vi "Config Timer App.vi"() -> ()   [LabVIEW 2017]
uses:
  subVIs/ModeEnumControl.ctl
  subVIs/AlarmElementControl.ctl
  subVIs/StateEnum.ctl
  subVIs/ModeEnum.ctl
  subVIs/AvailableEnum.ctl
  subVIs/StopWatchTimerStateEnum.ctl
  subVIs/AlarmConvertDirectionEnumControl.ctl
  subVIs/TimerActionEnumControlFGV.ctl
  <vilib>/Utility/file.llb/Write Delimited Spreadsheet (string).vi
  <vilib>/Utility/file.llb/Read Delimited Spreadsheet (string).vi
panel:
  out "Alarm Name":string
  out "Alarm":bool
  out "Path":path
  in  "stop":bool
  out "error out":errorcluster
  out "Clock":string
  in  "Mode Tabs":T1
  in  "Alarm Edit":bool
  in  "Alarm Save":bool
  in  "Alarm List":T2[](array[typedef])
  out "Timer Error":errorcluster
  out "Expired":bool
  out "Elasped Time":i32
  in  "Timer Start/Stop":bool
  in  "Duration (s)":i32
  in  "Lap":bool
  in  "Pause":bool
  out "SW Elapsed Time (s)":dbl format="%.1g"
  in  "SW Timer Start/Stop":bool
  out "SW Error":errorcluster
  # "(one at a time)"
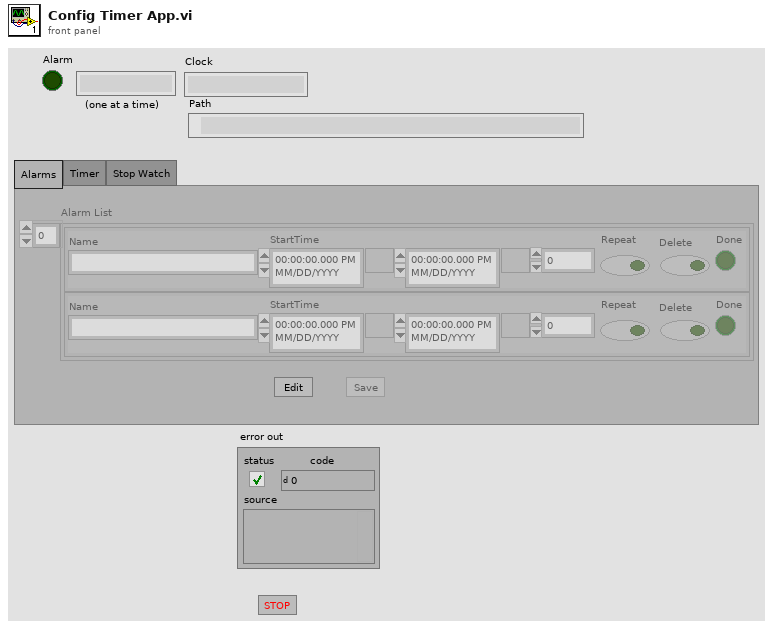
[diagram p1: front panel]
types:
  T1 = typedef "ModeEnumControl.ctl" = enum32{"Alarms", "Timer", "Stop Watch"}
  T2 = typedef "AlarmElementControl.ctl" = cluster{"Name":string, "StartTime ":timestamp, "End Time":timestamp, "Duration":i32, "Repeat":bool, "Delete":bool, "Done":bool}
  T3 = typedef "StopWatchTimerStateEnum.ctl" = enum16{"Start", "Idle", "Timing", "Lap", "Pause", "Stop"}
  T4 = cluster{"State":T3, "Duration":i32, "Start/Stop":bool, "Elapsed Time":dbl, "Expired":bool, "Pause":bool, "Lap":bool}
  T5 = cluster{"State":T3, "Duration":i32, "Start/Stop":bool, "Elapsed Time":i32, "Expired":bool}
  T6 = typedef "StateEnum.ctl" = enum16{"Startup", "Read Config", "Idle", "Timer"}
  T7 = typedef "ModeEnum.ctl" = enum16{"Alarms", "Timer"}
  T8 = typedef "AvailableEnum.ctl" = enum8{"Enabled", "Disabled", "Disabled and Grayed Out"}
  T9 = cluster{"State":T6, "Mode":T7, "Alarms":T2[], "Time":timestamp, "Alarm Edit Flag":bool, "Alarm List and Save Status":T8, "Alarm Edit Status":T8, "Path":path, "File":string, "Alarm Flag":bool, "Alarm Index":i32, "Alarmed Already":bool}
  T10 = typedef "TimerActionEnumControlFGV.ctl" = enum16{"Reset", "TimeQuery", "Pause", "Unpause"}
  T11 = typedef "AlarmConvertDirectionEnumControl.ctl" = enum16{"ToString", "ToCluster"}
  T12 = typedef "LVDateTimeRec.ctl" = cluster{"fractional second":dbl, "second":i32, "minute":i32, "hour":i32, "day of month":i32, "month":i32, "year":i32, "day of week":i32, "day of year":i32, "DST":i32}
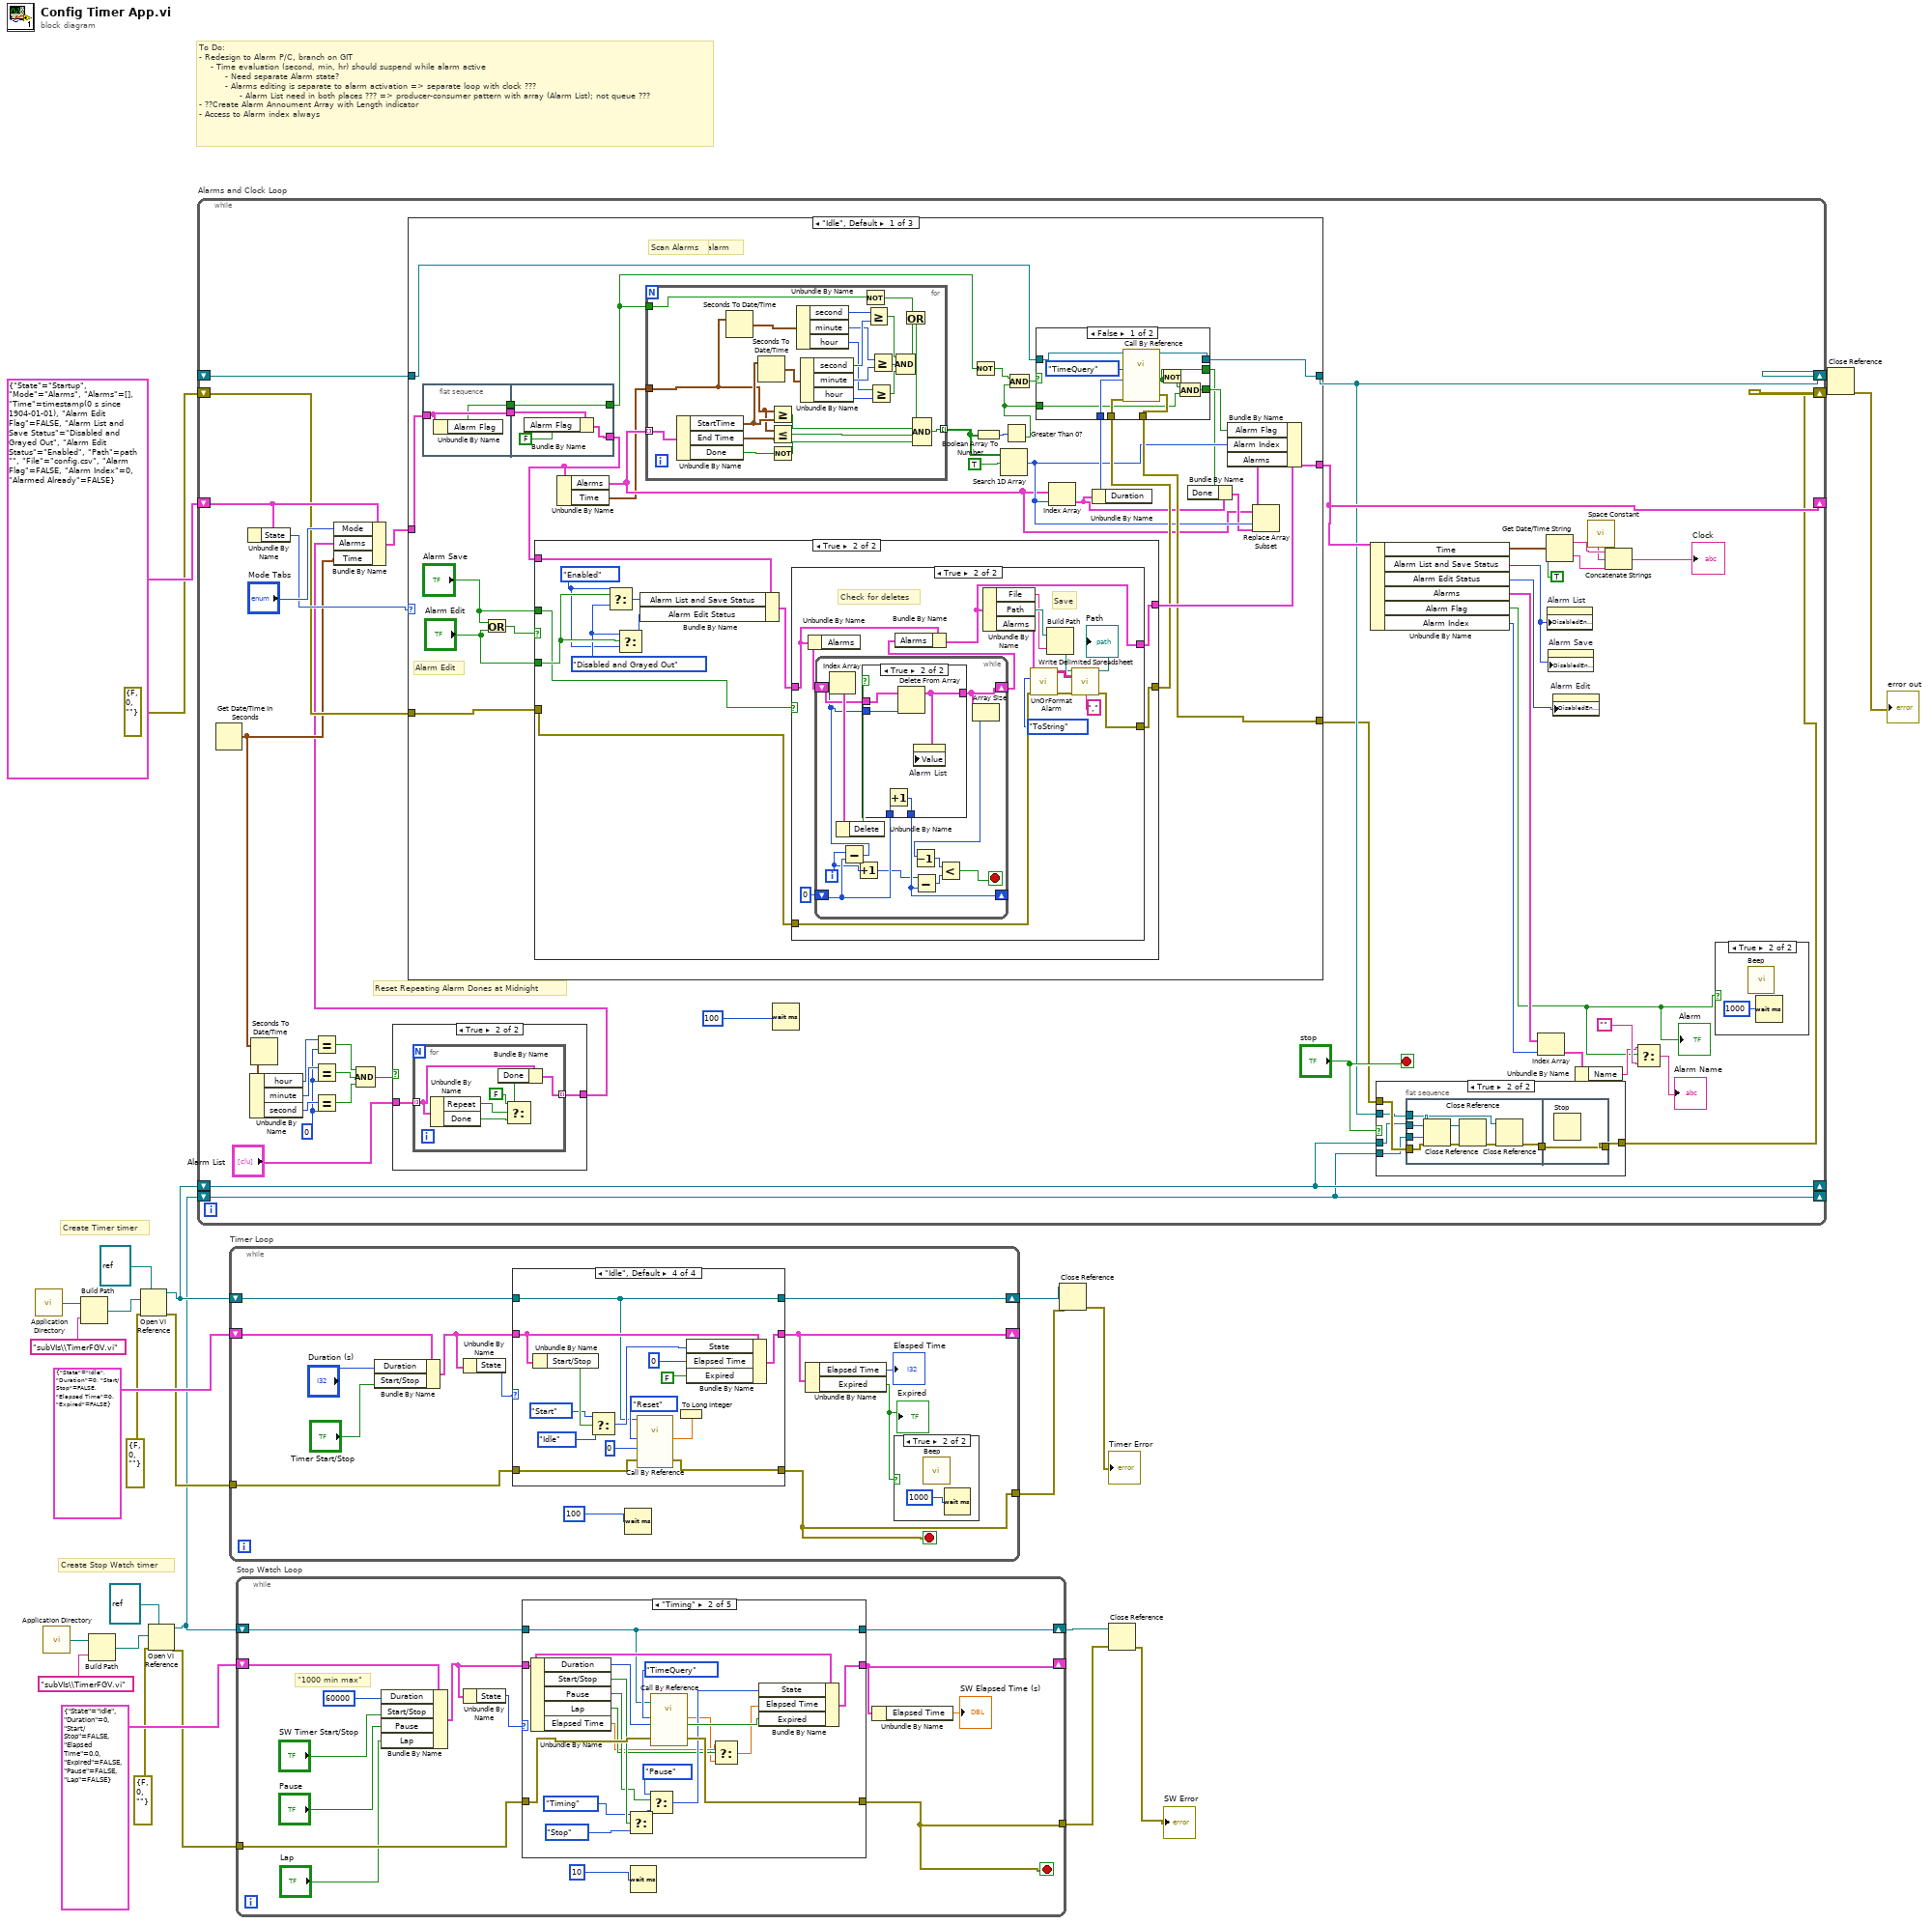
[diagram p0: block diagram]
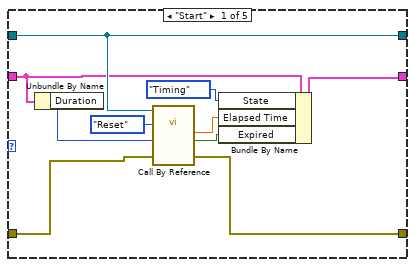
[diagram p2: hidden frame]
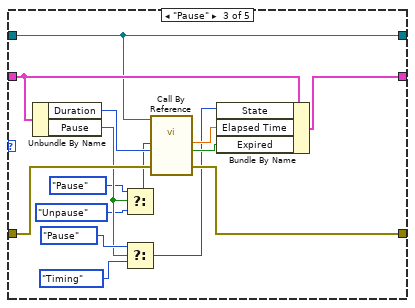
[diagram p3: hidden frame]
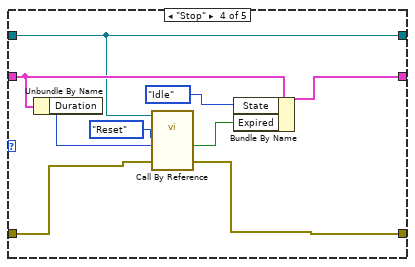
[diagram p4: hidden frame]
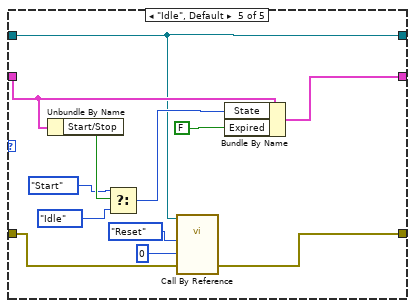
[diagram p5: hidden frame]
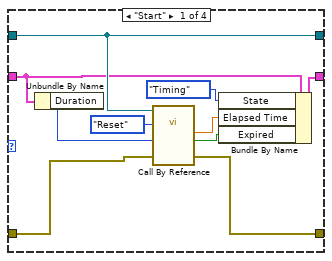
[diagram p7: hidden frame]
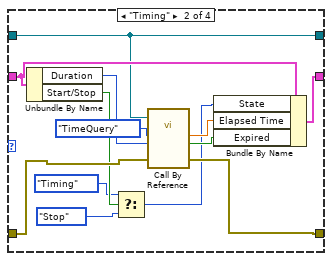
[diagram p8: hidden frame]
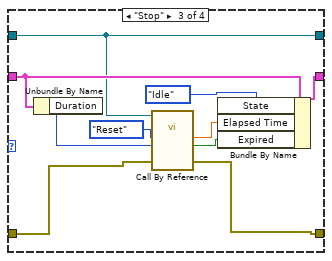
[diagram p9: hidden frame]
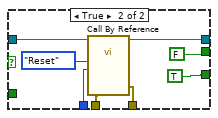
[diagram p13: hidden frame]
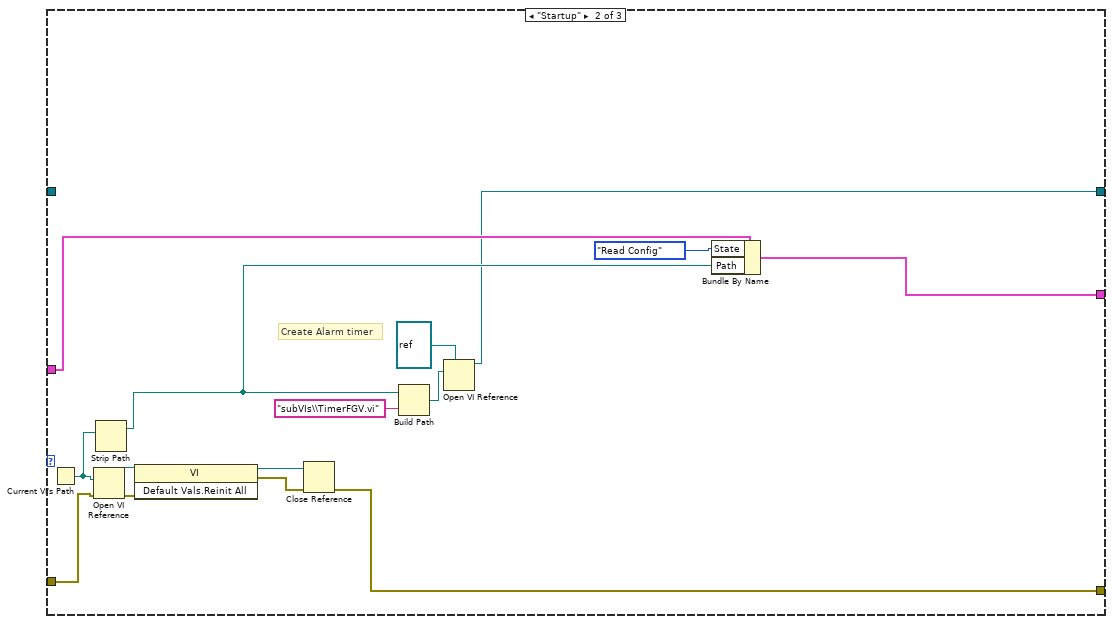
[diagram p17: hidden frame]
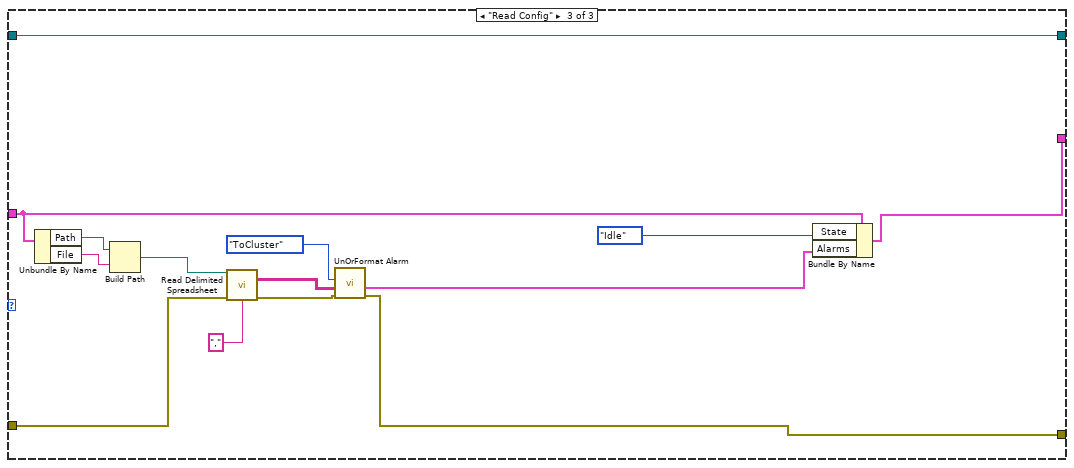
[diagram p18: hidden frame]
diagram:
  # "Create Stop Watch timer"
  # "Create Timer timer"
  # "To Do:\n- Redesign to Alarm P/C, branch on GIT\n    - Time evaluation (second, min, hr) should suspend while alarm active\n         - Need separate Alarm state?\n         - Alarms editing is separate to alarm activation => separate loop with clock ??? \n              - Alarm List need in both places ??? => producer-consumer pattern with array (Alarm List); not queue ???\n- ??Create Alarm Annoument Array with Length indicator\n- Access to Alarm index always"
  n1 = call <vilib>:"Application Directory.vi"() -> ("Application Directory"=w24:path)
  n2 = call <vilib>:"Application Directory.vi"() -> ("Application Directory"=w21:path)
  n3 = Build Path(base path=w24, name or relative path="subVIs\\TimerFGV.vi") -> (appended path=w18:path)
  n4 = Build Path(base path=w21, name or relative path="subVIs\\TimerFGV.vi") -> (appended path=w14:path)
  n5 = Open VI Reference(type specifier VI Refnum (for type only)=refnum<vi> refnum, vi path=w18, error in (no error)=errorcluster {"status"=FALSE, "code"=0, "source"=""} ("error constant")) -> (vi reference=w11:refnum<vi>, error out=w16:errorcluster)  [unwired: 3 in]
  n6 = Open VI Reference(type specifier VI Refnum (for type only)=refnum<vi> refnum, vi path=w14, error in (no error)=errorcluster {"status"=FALSE, "code"=0, "source"=""} ("error constant")) -> (vi reference=w10:refnum<vi>, error out=w12:errorcluster)  [unwired: 3 in]
  n7 = while "Alarms and Clock Loop" {
    shift-right: [w62] -> _
    shift-left: T9 {"State"=enum."Startup", "Mode"=enum."Alarms", "Alarms"=[], "Time"=timestamp(0 s since 1904-01-01), "Alarm Edit Flag"=FALSE, "Alarm List and Save Status"=enum."Disabled and Grayed Out", "Alarm Edit Status"=enum."Enabled", "Path"=path "", "File"="config.csv", "Alarm Flag"=FALSE, "Alarm Index"=0, "Alarmed Already"=FALSE} -> [w67]
    shift-right: [w29] -> w2
    shift-left: errorcluster {"status"=FALSE, "code"=0, "source"=""} ("error constant") -> [w64]
    shift-right: [w31] -> w4
    shift-left: _ -> [w51]
    shift-right: [w33] -> _
    shift-left: w11 -> [w33]
    shift-right: [w32] -> _
    shift-left: w10 -> [w32]
    stop <- "stop" stop-if-true
    w35 = 0
    # "Reset Repeating Alarm Dones at Midnight"
    n8 = Get Date/Time In Seconds() -> (seconds since 1Jan1904=w46:timestamp)
    n9 = Unbundle By Name(w67) -> ("State"=w65:T6)
    n10 = Seconds To Date/Time(time stamp (now)=w46) -> (date time rec=w45:T12)  [unwired: 1 in]
    n11 = Unbundle By Name(w45) -> ("hour"=w36:i32, "minute"=w44:i32, "second"=w43:i32)
    n12 = Equal?(x=w36, y=w35) -> (x = y?=w40:bool)
    n13 = Equal?(x=w44, y=w35) -> (x = y?=w41:bool)
    n14 = Equal?(x=w43, y=w35) -> (x = y?=w42:bool)
    n15 = Compound Arithmetic op=AND(w40, w41, w42) -> (w39:bool)
    n16 = case shown="True" w39 {
      tunnel: "Alarm List" -> [w85 w87]
      tunnel: [w85 w86] -> w37
      frame False {
      }
      frame True {
        n17 = for {
          tunnel: w87 -> [w92] mode=indexing
          tunnel: [w93] -> w86 mode=indexing
          n18 = Unbundle By Name(w92) -> ("Repeat"=w91:bool, "Done"=w89:bool)
          n19 = Select(t=FALSE, s=w91, f=w89) -> (s? t:f=w88:bool)
          n20 = Bundle By Name(cluster=w92, "Done"=w88) -> (w93:T2)
        }
      }
    }
    n21 = Bundle By Name(cluster=w67, "Mode"="Mode Tabs", "Alarms"=w37, "Time"=w46) -> (w63:T9)
    n22 = case shown="\"Idle\", Default" w65 {
      tunnel: w64 -> [w120 w235 w240]
      tunnel: [w110 w232 w239] -> w30
      tunnel: w63 -> [w109 w226 w249]
      tunnel: [w118 w230 w250] -> w62
      tunnel: [w113 w223 w238] -> w31
      tunnel: w51 -> [w114 _ w238]
      frame "Idle", Default {
        # "Find only first alarm"
        # "Alarm Edit"
        # "Scan Alarms"
        n23 = flat-sequence {
          tunnel: w109 -> [w143]
          tunnel: [w143] -> w107
          tunnel: [w142] -> w105
          tunnel: [w146] -> w108
          tunnel: w107 -> [w145]
          tunnel: [w144] -> w94
          tunnel: w105 -> [w144]
          frame #0 {
            n24 = Unbundle By Name(w143) -> ("Alarm Flag"=w142:bool)
          }
          frame #1 {
            n25 = Bundle By Name(cluster=w145, "Alarm Flag"=FALSE) -> (w146:T9)
          }
        }
        n26 = Or(x="Alarm Save", y="Alarm Edit") -> (x .or. y?=w123:bool)
        n27 = case shown="True" w123 {
          tunnel: w108 -> [w173 w184]
          tunnel: [w173 w174] -> w119
          tunnel: "Alarm Edit" -> [_ w183]
          tunnel: "Alarm Save" -> [_ w178]
          tunnel: w120 -> [w172 w176]
          tunnel: [w172 w175] -> w111
          frame False {
          }
          frame True {
            w181 = AvailableEnum."Disabled and Grayed Out" ("Enum")
            w180 = AvailableEnum."Enabled" ("Enum")
            n28 = Select(t=w180, s=w183, f=w181) -> (s? t:f=w182:T8)
            n29 = Select(t=w181, s=w183, f=w180) -> (s? t:f=w179:T8)
            n30 = Bundle By Name(cluster=w184, "Alarm List and Save Status"=w182, "Alarm Edit Status"=w179) -> (w177:T9)
            n31 = case shown="True" w178 {
              tunnel: w177 -> [w185 w191]
              tunnel: w176 -> [w186 w201]
              tunnel: [w186 w195] -> w175
              tunnel: [w185 w189] -> w174
              frame False {
              }
              frame True {
                # "Check for deletes"
                # "Save"
                n32 = Unbundle By Name(w191) -> ("Alarms"=w190:T2[])
                n33 = while {
                  shift-right: [w208] -> _
                  shift-left: 0 -> [w206]
                  shift-right: [w203] -> w187
                  shift-left: w190 -> [w213]
                  i -> [w205]
                  stop <- w210 stop-if-true
                  n34 = Subtract(x=w205, y=w206) -> (x-y=w209:i32)
                  n35 = Index Array(array=w213, index=w209) -> (element=w215:T2)
                  n36 = Unbundle By Name(w215) -> ("Delete"=w214:bool)
                  n37 = Increment(x=w205) -> (x+1=w204:i32)
                  n38 = case shown="True" w214 {
                    tunnel: w213 -> [w217 w222]
                    tunnel: w209 -> [_ w219]
                    tunnel: [w217 w218] -> w203
                    tunnel: w206 -> [w216 w221]
                    tunnel: [w216 w220] -> w208
                    frame False {
                    }
                    frame True {
                      n39 = Increment(x=w221) -> (x+1=w220:i32)
                      n40 = Delete From Array(array=w222, index=w219) -> (array with subset deleted=w218:T2[])  [unwired: 1 in, 1 out]
                      n41 = property on="Alarm List" class="Arr (strict)"("Value"=w218) -> ()  [unwired: 2 in, 2 out]
                    }
                  }
                  n42 = Subtract(x=w204, y=w208) -> (x-y=w207:i32)
                  n43 = Array Size(array=w203) -> (size(s)=w212:i32)
                  n44 = Decrement(x=w212) -> (x-1=w211:i32)
                  n45 = Less?(x=w211, y=w207) -> (x < y?=w210:bool)
                }
                n46 = Bundle By Name(cluster=w191, "Alarms"=w187) -> (w189:T9)
                n47 = Unbundle By Name(w189) -> ("File"=w192:string, "Path"=w197:path, "Alarms"=w200:T2[])
                n48 = call "UnOrFormat Alarm.vi"("error in (no error)"=w201, "Direction"=AlarmConvertDirectionEnumControl."ToString", "Alarms List In"=w200) -> ("error out"=w202:errorcluster, "Alarm String Array Out"=w198:string[][])  [unwired: 6 in, 1 out]
                n49 = Build Path(base path=w197, name or relative path=w192) -> (appended path=w196:path)
                n50 = call-poly <vilib>:"Write Delimited Spreadsheet.vi"("file path (dialog if empty)"=w196, "2D data"=w198, "error in (no error)"=w202, "delimiter (\\t)"=",") -> ("new file path (Not A Path if cancelled)"=→"Path":path, "error out"=w195:errorcluster)  [unwired: 10 in]
              }
            }
          }
        }
        n51 = Unbundle By Name(w108) -> ("Alarms"=w98:T2[], "Time"=w95:timestamp)
        n52 = for {
          tunnel: w98 -> [w166] mode=indexing
          tunnel: [w169] -> w115 mode=indexing
          tunnel: w95 -> [w156]
          tunnel: w94 -> [w154]
          n53 = Unbundle By Name(w166) -> ("StartTime"=w165:timestamp, "End Time"=w155:timestamp, "Done"=w168:bool)
          n54 = Seconds To Date/Time(time stamp (now)=w156) -> (date time rec=w164:T12)  [unwired: 1 in]
          n55 = Seconds To Date/Time(time stamp (now)=w165) -> (date time rec=w163:T12)  [unwired: 1 in]
          n56 = Greater Or Equal?(x=w156, y=w165) -> (x >= y?=w171:bool)
          n57 = Less Or Equal?(x=w156, y=w155) -> (x <= y?=w170:bool)
          n58 = Not(x=w168) -> (.not. x?=w167:bool)
          n59 = Unbundle By Name(w164) -> ("second"=w162:i32, "minute"=w160:i32, "hour"=w158:i32)
          n60 = Unbundle By Name(w163) -> ("second"=w161:i32, "minute"=w159:i32, "hour"=w157:i32)
          n61 = Not(x=w154) -> (.not. x?=w150:bool)
          n62 = Greater Or Equal?(x=w162, y=w161) -> (x >= y?=w152:bool)
          n63 = Greater Or Equal?(x=w158, y=w157) -> (x >= y?=w151:bool)
          n64 = Greater Or Equal?(x=w160, y=w159) -> (x >= y?=w153:bool)
          n65 = Compound Arithmetic op=AND(w152, w153, w151) -> (w149:bool)
          n66 = Or(x=w150, y=w149) -> (x .or. y?=w148:bool)
          n67 = Compound Arithmetic op=AND(w148, w171, w170, w167) -> (w169:bool)
        }
        n68 = Not(x=w94) -> (.not. x?=w104:bool)
        n69 = Boolean Array To Number(Boolean array=w115) -> (number=w117:u32)
        n70 = Search 1D Array(1D array=w115, element=TRUE) -> (index of element=w100:i32)  [unwired: 1 in]
        n71 = Greater Than 0?(x=w117) -> (x > 0?=w102:bool)
        n72 = And(x=w104, y=w102) -> (x .and. y?=w103:bool)
        n73 = Index Array(array=w98, index=w100) -> (element=w101:T2)
        n74 = Unbundle By Name(w101) -> ("Duration"=w112:i32)
        n75 = case shown="False" w103 {
          tunnel: w114 -> [w132 w141]
          tunnel: [w128 w140] -> w113
          tunnel: w112 -> [w131 w139]
          tunnel: w111 -> [w130 w138]
          tunnel: [w129 w137] -> w110
          tunnel: [w125 TRUE] -> w106
          tunnel: w102 -> [w126 _]
          tunnel: [w124 FALSE] -> w96
          frame False {
            n76 = call-by-ref "?"(reference=w132, "error in (no error)"=w130, "Target (s)"=w131, "Action"=TimerActionEnumControlFGV."TimeQuery") -> (reference out=w128:refnum<vi>, "error out"=w129:errorcluster, "Elapsed"=w124:bool)  [unwired: 7 in, 2 out]
            n77 = Not(x=w124) -> (.not. x?=w127:bool)
            n78 = And(x=w127, y=w126) -> (x .and. y?=w125:bool)
          }
          frame True {
            n79 = call-by-ref "?"(reference=w141, "error in (no error)"=w138, "Target (s)"=w139, "Action"=TimerActionEnumControlFGV."Reset") -> (reference out=w140:refnum<vi>, "error out"=w137:errorcluster)  [unwired: 7 in, 3 out]
          }
        }
        n80 = Bundle By Name(cluster=w101, "Done"=w96) -> (w99:T2)
        n81 = Replace Array Subset(array=w98, new element=w99, index=w100) -> (w97:T2[])
        n82 = Bundle By Name(cluster=w119, "Alarm Flag"=w106, "Alarm Index"=w100, "Alarms"=w97) -> (w118:T9)
      }
      frame "Startup" {
        # "Create Alarm timer"
        n83 = Current VI's Path() -> (path=w229:path)
        n84 = Open VI Reference(vi path=w229, error in (no error)=w235) -> (vi reference=w236:refnum<vi>, error out=w237:errorcluster)  [unwired: 4 in]
        n85 = Strip Path(path=w229) -> (stripped path=w228:path)  [unwired: 1 out]
        n86 = invoke class="VI" method="Default Vals.Reinit All"(reference=w236, error in=w237) -> (reference out=w234:refnum<vi>, error out=w233:errorcluster)  [unwired: 1 in, 1 out]
        n87 = Close Reference(reference=w234, error in (no error)=w233) -> (error out=w232:errorcluster)
        n88 = Build Path(base path=w228, name or relative path="subVIs\\TimerFGV.vi") -> (appended path=w225:path)
        n89 = Open VI Reference(type specifier VI Refnum (for type only)=refnum<vi> refnum, vi path=w225) -> (vi reference=w223:refnum<vi>)  [unwired: 4 in, 1 out]
        n90 = Bundle By Name(cluster=w226, "State"=StateEnum."Read Config", "Path"=w228) -> (w230:T9)
      }
      frame "Read Config" {
        n91 = Unbundle By Name(w249) -> ("Path"=w248:path, "File"=w247:string)
        n92 = Build Path(base path=w248, name or relative path=w247) -> (appended path=w246:path)
        n93 = call-poly <vilib>:"Read Delimited Spreadsheet.vi"("file path (dialog if empty)"=w246, "error in (no error)"=w240, "delimiter (\\t)"=",") -> ("all rows"=w244:string[][], "error out"=w241:errorcluster)  [unwired: 7 in, 4 out]
        n94 = call "UnOrFormat Alarm.vi"("error in (no error)"=w241, "Alarm String Array In"=w244, "Direction"=AlarmConvertDirectionEnumControl."ToCluster") -> ("error out"=w239:errorcluster, "Alarms List Out"=w242:T2[])  [unwired: 6 in, 1 out]
        n95 = Bundle By Name(cluster=w249, "State"=StateEnum."Idle", "Alarms"=w242) -> (w250:T9)
      }
    }
    n96 = Wait (ms)(milliseconds to wait=u32 100) -> ()  [unwired: 1 out]
    n97 = Unbundle By Name(w62) -> ("Time"=w61:timestamp, "Alarm List and Save Status"=w55:T8, "Alarm Edit Status"=w47:T8, "Alarms"=w54:T2[], "Alarm Flag"=w28:bool, "Alarm Index"=w53:i32)
    "Alarm" <- w28
    n98 = case shown="True" "stop" {
      tunnel: w33 -> [_ w74]
      tunnel: w32 -> [_ w73]
      tunnel: w31 -> [_ w75]
      tunnel: w30 -> [w70 w76]
      tunnel: [w70 w72] -> w29
      frame False {
      }
      frame True {
        n99 = flat-sequence {
          tunnel: w76 -> [w82]
          tunnel: w75 -> [w79]
          tunnel: w74 -> [w81]
          tunnel: w73 -> [w83]
          tunnel: [w77] -> w71
          tunnel: [w84] -> w72
          tunnel: w71 -> [w84]
          frame #0 {
            n100 = Close Reference(reference=w83, error in (no error)=w82) -> (error out=w80:errorcluster)
            n101 = Close Reference(reference=w81, error in (no error)=w80) -> (error out=w78:errorcluster)
            n102 = Close Reference(reference=w79, error in (no error)=w78) -> (error out=w77:errorcluster)
          }
          frame #1 {
            n103 = Stop() -> ()  [unwired: 1 in]
          }
        }
      }
    }
    n104 = Index Array(array=w54, index=w53) -> (element=w52:T2)
    n105 = Get Date/Time String(seconds (now)=w61, want seconds? (F)=TRUE) -> (date string=w59:string, time string=w57:string)  [unwired: 1 in]
    n106 = property on="Alarm List" class="Arr (strict)"("DisabledEnum"=w55) -> ()  [unwired: 2 in, 2 out]
    n107 = property on="Alarm Save" class="Bool"("DisabledEnum"=w55) -> ()  [unwired: 2 in, 2 out]
    n108 = property on="Alarm Edit" class="Bool"("DisabledEnum"=w47) -> ()  [unwired: 2 in, 2 out]
    n109 = Unbundle By Name(w52) -> ("Name"=w49:string)
    n110 = call <vilib>:"Space Constant.vi"() -> ("String"=w58:string)
    n111 = Concatenate Strings(w59, w58, w57) -> (→"Clock":string)
    n112 = Select(t=w49, s=w28, f="") -> (s? t:f=→"Alarm Name":string)
    n113 = case shown="True" w28 {
      frame False {
      }
      frame True {
        n114 = call <vilib>:"Beep.vi"() -> ()  [unwired: 12 in]
        n115 = Wait (ms)(milliseconds to wait=u32 1000) -> ()  [unwired: 1 out]
      }
    }
  }
  n116 = while "Timer Loop" {
    shift-right: [w257] -> _
    shift-left: T5 {"State"=enum."Idle", "Duration"=0, "Start/Stop"=FALSE, "Elapsed Time"=0, "Expired"=FALSE} -> [w254]
    tunnel: w16 -> [w260]
    shift-right: [w258] -> w6
    shift-left: w11 -> [w259]
    tunnel: [w253] -> w5
    stop <- w253 stop-if-true
    n117 = Bundle By Name(cluster=w254, "Duration"="Duration (s)", "Start/Stop"="Timer Start/Stop") -> (w255:T5)
    n118 = Unbundle By Name(w255) -> ("State"=w263:T3)
    n119 = case shown="\"Idle\", Default" w263 {
      tunnel: w255 -> [w270 w284 w293 w311]
      tunnel: [w269 w280 w289 w310] -> w257
      tunnel: w260 -> [w274 w283 w292 w304]
      tunnel: [w273 w282 w291 w303] -> w253
      tunnel: w259 -> [w275 w281 w290 w300]
      tunnel: [w275 w281 w290 w300] -> w258
      frame "Start" {
        n120 = Unbundle By Name(w270) -> ("Duration"=w272:i32)
        n121 = call-by-ref "?"(reference=w275, "error in (no error)"=w274, "Target (s)"=w272, "Action"=TimerActionEnumControlFGV."Reset") -> ("error out"=w273:errorcluster, "Elapsed"=w267:bool, "Time"=w268:dbl)  [unwired: 7 in, 2 out]
        n122 = Bundle By Name(cluster=w270, "State"=StopWatchTimerStateEnum."Timing" ("Enum"), "Elapsed Time"=w268, "Expired"=w267) -> (w269:T5)
      }
      frame "Timing" {
        n123 = Unbundle By Name(w284) -> ("Duration"=w286:i32, "Start/Stop"=w279:bool)
        n124 = Select(t=StopWatchTimerStateEnum."Timing" ("Enum"), s=w279, f=StopWatchTimerStateEnum."Stop" ("Enum")) -> (s? t:f=w276:T3)
        n125 = call-by-ref "?"(reference=w281, "error in (no error)"=w283, "Target (s)"=w286, "Action"=TimerActionEnumControlFGV."TimeQuery") -> ("error out"=w282:errorcluster, "Elapsed"=w288:bool, "Time"=w287:dbl)  [unwired: 7 in, 2 out]
        n126 = Bundle By Name(cluster=w284, "State"=w276, "Elapsed Time"=w287, "Expired"=w288) -> (w280:T5)
      }
      frame "Stop" {
        n127 = Unbundle By Name(w293) -> ("Duration"=w296:i32)
        n128 = call-by-ref "?"(reference=w290, "error in (no error)"=w292, "Target (s)"=w296, "Action"=TimerActionEnumControlFGV."Reset") -> ("error out"=w291:errorcluster, "Elapsed"=w298:bool, "Time"=w297:dbl)  [unwired: 7 in, 2 out]
        n129 = Bundle By Name(cluster=w293, "State"=StopWatchTimerStateEnum."Idle" ("Enum"), "Elapsed Time"=w297, "Expired"=w298) -> (w289:T5)
      }
      frame "Idle", Default {
        n130 = Unbundle By Name(w311) -> ("Start/Stop"=w309:bool)
        n131 = Select(t=StopWatchTimerStateEnum."Start" ("Enum"), s=w309, f=StopWatchTimerStateEnum."Idle" ("Enum")) -> (s? t:f=w306:T3)
        n132 = call-by-ref "?"(reference=w300, "error in (no error)"=w304, "Target (s)"=0, "Action"=TimerActionEnumControlFGV."Reset") -> ("error out"=w303:errorcluster, "Time"=w302:dbl)  [unwired: 7 in, 3 out]
        n133 = To Long Integer(number=w302) -> ()  [unwired: 1 out]
        n134 = Bundle By Name(cluster=w311, "State"=w306, "Elapsed Time"=0, "Expired"=FALSE) -> (w310:T5)
      }
    }
    n135 = Wait (ms)(milliseconds to wait=u32 100) -> ()  [unwired: 1 out]
    n136 = Unbundle By Name(w257) -> ("Elapsed Time"=→"Elasped Time":i32, "Expired"=w252:bool)
    "Expired" <- w252
    n137 = case shown="True" w252 {
      frame False {
      }
      frame True {
        n138 = call <vilib>:"Beep.vi"() -> ()  [unwired: 12 in]
        n139 = Wait (ms)(milliseconds to wait=1000) -> ()  [unwired: 1 out]
      }
    }
  }
  n140 = while "Stop Watch Loop" {
    shift-right: [w318] -> _
    shift-left: T4 {"State"=enum."Idle", "Duration"=0, "Start/Stop"=FALSE, "Elapsed Time"=0.0, "Expired"=FALSE, "Pause"=FALSE, "Lap"=FALSE} -> [w323]
    tunnel: w12 -> [w322]
    shift-right: [w320] -> w9
    shift-left: w10 -> [w321]
    tunnel: [w319] -> w8
    stop <- w319 stop-if-true
    # "\"1000 min max\""
    n141 = Bundle By Name(cluster=w323, "Duration"=60000, "Start/Stop"="SW Timer Start/Stop", "Pause"="Pause", "Lap"="Lap") -> (w316:T4)
    n142 = Unbundle By Name(w316) -> ("State"=w325:T3)
    n143 = case shown="\"Timing\"" w325 {
      tunnel: w316 -> [w331 w352 w367 w375 w390]
      tunnel: [w330 w348 w360 w371 w389] -> w318
      tunnel: w322 -> [w335 w351 w365 w374 w384]
      tunnel: [w334 w350 w364 w373 w383] -> w319
      tunnel: w321 -> [w336 w349 w366 w372 w382]
      tunnel: [w336 w349 w366 w372 w382] -> w320
      frame "Start" {
        n144 = Unbundle By Name(w331) -> ("Duration"=w333:i32)
        n145 = call-by-ref "?"(reference=w336, "error in (no error)"=w335, "Target (s)"=w333, "Action"=TimerActionEnumControlFGV."Reset") -> ("error out"=w334:errorcluster, "Elapsed"=w328:bool, "Time"=w329:dbl)  [unwired: 7 in, 2 out]
        n146 = Bundle By Name(cluster=w331, "State"=StopWatchTimerStateEnum."Timing" ("Enum"), "Elapsed Time"=w329, "Expired"=w328) -> (w330:T4)
      }
      frame "Timing" {
        n147 = Unbundle By Name(w352) -> ("Duration"=w354:i32, "Start/Stop"=w347:bool, "Pause"=w342:bool, "Lap"=w340:bool, "Elapsed Time"=w339:dbl)
        n148 = Select(t=StopWatchTimerStateEnum."Timing" ("Enum"), s=w347, f=StopWatchTimerStateEnum."Stop" ("Enum")) -> (s? t:f=w344:T3)
        n149 = Select(t=StopWatchTimerStateEnum."Pause" ("Enum"), s=w342, f=w344) -> (s? t:f=w343:T3)
        n150 = call-by-ref "?"(reference=w349, "error in (no error)"=w351, "Target (s)"=w354, "Action"=TimerActionEnumControlFGV."TimeQuery") -> ("error out"=w350:errorcluster, "Elapsed"=w355:bool, "Time"=w338:dbl)  [unwired: 7 in, 2 out]
        n151 = Select(t=w339, s=w340, f=w338) -> (s? t:f=w337:dbl)
        n152 = Bundle By Name(cluster=w352, "State"=w343, "Elapsed Time"=w337, "Expired"=w355) -> (w348:T4)
      }
      frame "Pause" {
        n153 = Unbundle By Name(w367) -> ("Duration"=w368:i32, "Pause"=w359:bool)
        n154 = Select(t=TimerActionEnumControlFGV."Pause" ("Action"), s=w359, f=TimerActionEnumControlFGV."Unpause" ("Action")) -> (s? t:f=w356:T10)
        n155 = Select(t=StopWatchTimerStateEnum."Pause" ("Enum"), s=w359, f=StopWatchTimerStateEnum."Timing" ("Enum")) -> (s? t:f=w361:T3)
        n156 = call-by-ref "?"(reference=w366, "error in (no error)"=w365, "Target (s)"=w368, "Action"=w356) -> ("error out"=w364:errorcluster, "Elapsed"=w370:bool, "Time"=w369:dbl)  [unwired: 7 in, 2 out]
        n157 = Bundle By Name(cluster=w367, "State"=w361, "Elapsed Time"=w369, "Expired"=w370) -> (w360:T4)
      }
      frame "Stop" {
        n158 = Unbundle By Name(w375) -> ("Duration"=w378:i32)
        n159 = call-by-ref "?"(reference=w372, "error in (no error)"=w374, "Target (s)"=w378, "Action"=TimerActionEnumControlFGV."Reset") -> ("error out"=w373:errorcluster, "Elapsed"=w379:bool)  [unwired: 7 in, 3 out]
        n160 = Bundle By Name(cluster=w375, "State"=StopWatchTimerStateEnum."Idle" ("Enum"), "Expired"=w379) -> (w371:T4)
      }
      frame "Idle", Default {
        n161 = Unbundle By Name(w390) -> ("Start/Stop"=w388:bool)
        n162 = Select(t=StopWatchTimerStateEnum."Start" ("Enum"), s=w388, f=StopWatchTimerStateEnum."Idle" ("Enum")) -> (s? t:f=w385:T3)
        n163 = call-by-ref "?"(reference=w382, "error in (no error)"=w384, "Target (s)"=0, "Action"=TimerActionEnumControlFGV."Reset") -> ("error out"=w383:errorcluster)  [unwired: 7 in, 4 out]
        n164 = Bundle By Name(cluster=w390, "State"=w385, "Expired"=FALSE) -> (w389:T4)
      }
    }
    n165 = Wait (ms)(milliseconds to wait=u32 10) -> ()  [unwired: 1 out]
    n166 = Unbundle By Name(w318) -> ("Elapsed Time"=→"SW Elapsed Time (s)":dbl)
  }
  n167 = Close Reference(reference=w6, error in (no error)=w5) -> (error out=→"Timer Error":errorcluster)
  n168 = Close Reference(reference=w9, error in (no error)=w8) -> (error out=→"SW Error":errorcluster)
  n169 = Close Reference(reference=w4, error in (no error)=w2) -> (error out=→"error out":errorcluster)
